vi "CCL.vi"(0 "System no.":i32=1 min=1 max=4 step=1, 2 "Command level":i32, 3 "Password":string, 5 "error in":errorcluster) -> (14 "Controller error":bool, 19 "error out":errorcluster)   [LabVIEW 2013]
doc: "If password is correct, this vi sets the command level of the controller and queries ERR?. Controller error is TRUE if selected system report error code not equal to zero. Use \"HLP?.vi\" to determine which commands are available in the current command level.\n\nValid for E-517, E-709, E-710, E-712, E-725, E-753, E-755\n\nE-517, E-709, E-710, E-712, E-725, E-753, E-755, F-206, M-8X0: Command level can be 0 (only commands needed for normal operation are available) or 1 (all commands from command level 0 plus special commands for advanced users are available). Password for CCL 1 is \"ADVANCED\".\n\nF-206: Check HLP?/HELP answer to find out if CCL is supported. Only for GCS syntax version = GCS 2.0 or higher (check with CSV?.vi. If CSV?.vi is not supported, syntax version is GCS 1.0).\n\nM-8X0: Check HLP?/HELP answer to find out if CCL is supported. Only for GCS syntax version = GCS 2.0 or higher (check with CSV?.vi. If CSV?.vi is not supported, syntax version is GCS 1.0)."
panel:
  # "If password is correct, this vi sets the command level of the controller and \nqueries ERR?. See VI description for available levels. Use \"HLP?.vi\" to determine\nwhich commands are available in the current command level."
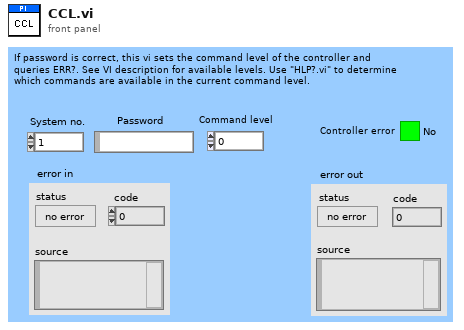
[diagram p1: front panel]
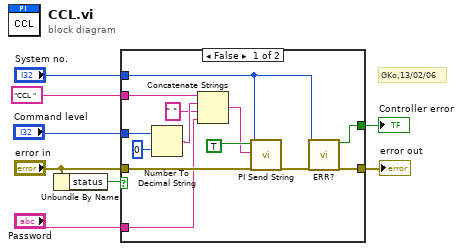
[diagram p0: block diagram]
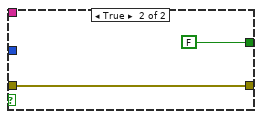
[diagram p2: hidden frame]
diagram:
  # "GKo,13/02/06"
  n1 = Unbundle By Name("error in") -> ("status"=w2:bool)
  n2 = case shown="False" w2 {
    tunnel: [w21 w22] -> w8
    tunnel: "CCL " -> [w20 _]
    tunnel: "System no." -> [w18 _]
    tunnel: "Password" -> [w10 _]
    tunnel: [w16 FALSE ("Controller error")] -> w4
    tunnel: "error in" -> [w15 w22]
    tunnel: "Command level" -> [w14 _]
    frame False {
      n3 = Number To Decimal String(number=w14, width (-)=i16 0) -> (decimal integer string=w12:string)
      n4 = Concatenate Strings(w20, w12, " " ("Substring"), w10) -> (w17:string)
      n5 = call "PI Send String.vi"("System no."=w18, "String to send"=w17, "Attach termination char.?"=TRUE ("Attach Linefeed?"), "error in"=w15) -> ("error out"=w9:errorcluster)  [unwired: 15 in]
      n6 = call "ERR?.vi"("System no."=w18, "error in"=w9) -> ("Controller error"=w16:bool, "error out"=w21:errorcluster)  [unwired: 16 in]
    }
    frame True {
    }
  }
  "error out" <- w8
  "Controller error" <- w4
